vi "remove-br-.vi"() -> ()   [LabVIEW 2018]
panel:
  out "result string":string
  out "x = y?":bool
  out "concatenated string":string
  out "text":string
  in  "file (use dialog)":path=path "D:/Users/Nano/Documents/GitHub/manga/LN/Overload/Vol15/Overload_Vol15_Ch0.html"
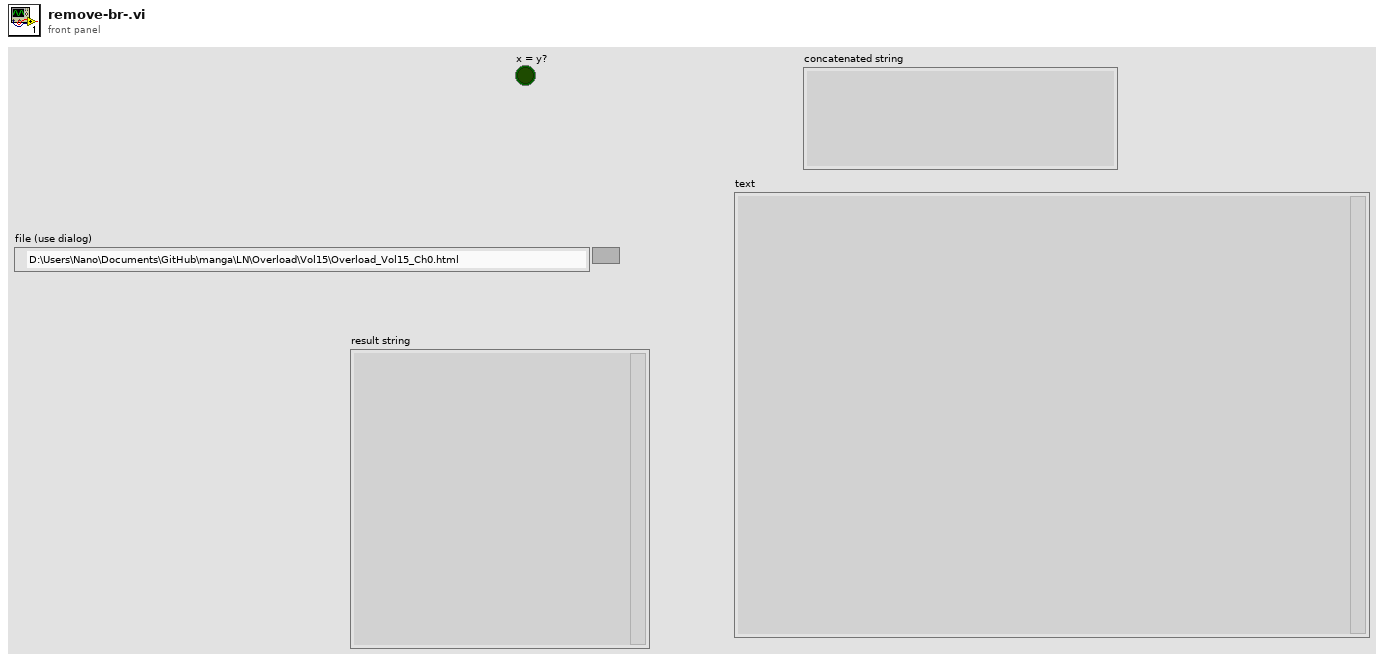
[diagram p1: front panel]
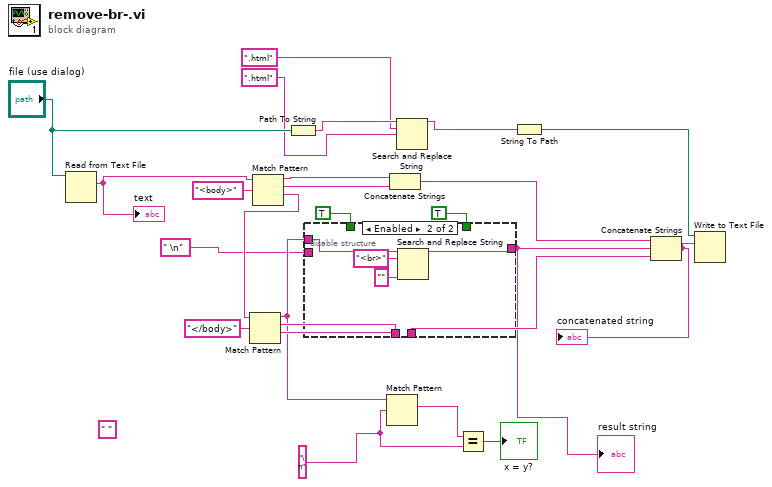
[diagram p0: block diagram]
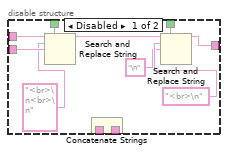
[diagram p2: hidden frame]
diagram:
  (unwired) " " ("search string")
  w5 = "\n" ("search string")
  n1 = Read from Text File(file (use dialog)="file (use dialog)") -> (text=w25:string)  [unwired: 3 in, 3 out]
  "text" <- w25
  n2 = Match Pattern(string=w25, regular expression="<body>") -> (before substring=w21:string, match substring=w20:string, after substring=w15:string)  [unwired: 1 in, 1 out]
  n3 = Match Pattern(string=w15, regular expression="</body>") -> (before substring=w3:string, match substring=w19:string, after substring=w18:string)  [unwired: 1 in, 1 out]
  n4 = Path To String(path="file (use dialog)") -> (string=w12:string)
  n5 = disable-structure shown="Enabled" {
    disable-tunnel: w19 -> [w37 _]
    disable-tunnel: w18 -> [w36 _]
    disable-tunnel: [w35 _] -> w16
    disable-tunnel: [w34 w41] -> w14
    disable-tunnel: TRUE ("replace all? (F)") -> [w33 _]
    disable-tunnel: w3 -> [w32 w40]
    disable-tunnel: TRUE ("replace all? (F)") -> [w30 _]
    disable-tunnel: " \n" ("search string") -> [w29 _]
    frame Disabled {
      n6 = Search and Replace String(replace all?=w30, input string=w32, search string="<br>\n<br>\n" ("replace string (\"\")"), replace string=w29) -> (result string=w31:string)  [unwired: 4 in, 3 out]
      n7 = Concatenate Strings(w37, w36) -> (w35:string)
      n8 = Search and Replace String(replace all?=w33, input string=w31, search string="<br>\n" ("replace string (\"\")"), replace string="\n" ("search string")) -> (result string=w34:string)  [unwired: 4 in, 3 out]
    }
    frame Enabled {
      n9 = Search and Replace String(input string=w40, search string="<br>", replace string="" ("replace string (\"\")")) -> (result string=w41:string)  [unwired: 5 in, 3 out]
    }
  }
  "result string" <- w14
  n10 = Match Pattern(string=w3, regular expression=w5) -> (match substring=w6:string)  [unwired: 1 in, 3 out]
  n11 = Concatenate Strings(w21, w20) -> (w17:string)
  n12 = Search and Replace String(input string=w12, search string=".html", replace string=".html" ("replace string (\"\")")) -> (result string=w11:string)  [unwired: 5 in, 3 out]
  n13 = Equal?(x=w6, y=w5) -> (x = y?=→"x = y?":bool)
  n14 = String To Path(string=w11) -> (path=w8:path)
  n15 = Concatenate Strings(w17, w14, w16) -> (w13:string)
  "concatenated string" <- w13
  n16 = Write to Text File(file (use dialog)=w8, text=w13) -> ()  [unwired: 2 in, 3 out]
